vi "Bodies_GenDH.vi"(4 "Mass(kg)":dbl, 6 "CoM_Pos":T2={"Coord4"=[0.0, 0.0, 0.0, 1.0], "ID"=0}, 7 "Unknown(theta)":enum16{"Theta", "Alpha", "a", "d"}(ring), 8 "theta(0)":dbl, 9 "alpha(0)":dbl, 10 "d(0)":dbl, 11 "a(0)":dbl) -> (3 "cluster":T3)   [LabVIEW 2015, in "Bodies.lvclass"]
uses:
  Bodies.lvclass
  PointOnBody.ctl
  DH_parameters.ctl
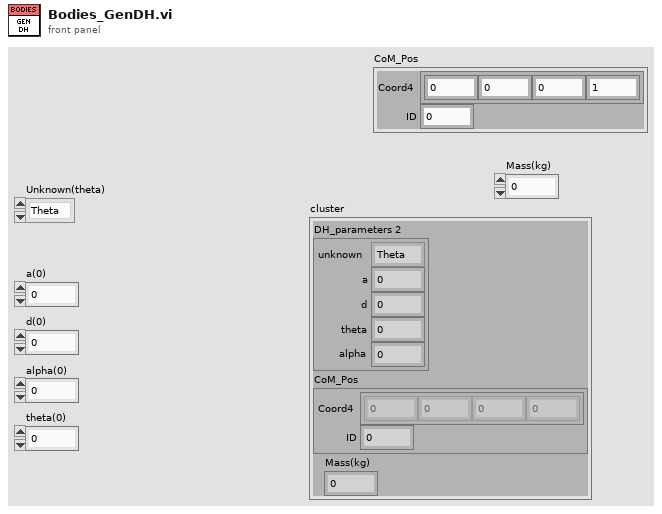
[diagram p1: front panel]
types:
  T1 = typedef "Bodies.lvclass/DH_parameters.ctl" = cluster{"unknown":enum16{"Theta", "Alpha", "a", "d"}, "a":dbl, "d":dbl, "alpha":dbl, "theta":dbl}
  T2 = typedef "Bodies.lvclass/PointOnBody.ctl" = cluster{"Coord4":dbl[], "ID":i32}
  T3 = cluster{"DH_parameters 2":T1, "CoM_Pos":T2, "Mass(kg)":dbl}
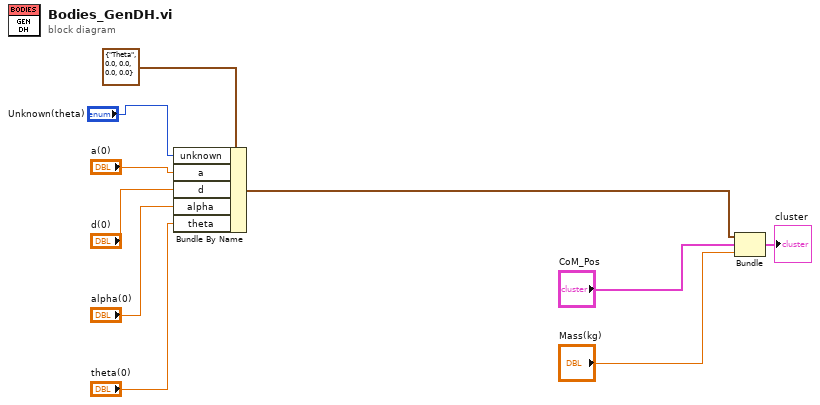
[diagram p0: block diagram]
diagram:
  n1 = Bundle By Name(cluster=T1 {"unknown"=enum."Theta", "a"=0.0, "d"=0.0, "alpha"=0.0, "theta"=0.0} ("DH_parameters 2"), "unknown"="Unknown(theta)", "a"="a(0)", "d"="d(0)", "alpha"="alpha(0)", "theta"="theta(0)") -> (w2:T1)
  n2 = Bundle("DH_parameters 2"=w2, "CoM_Pos"="CoM_Pos", "Mass(kg)"="Mass(kg)") -> (→"cluster":T3)  [unwired: 1 in]
